vi "Get Property Values (Date Property).vi"(1 "data type":timestamp[](array[timestamp]), 5 "property":T2 {"data type" items=["Unknown"=0, "String"=23, "I32"=3, "I64"=4, "DBL"=10, "Time stamp"=30]; "object type" items=["File", "Channel Group", "Channel"]}, 7 "result references":T1[](array[typedef]), 11 "error in (no error)":errorcluster) -> (6 "property values":timestamp[](array[timestamp]), 8 "result references out":T1[](array[typedef]), 15 "error out":errorcluster)   [LabVIEW 2020, in "NI_DataFinder.lvlib"]
doc: "Determines from the result references the values of a time/date property."
uses:
  <vilib>/DataFinder/NI_DataFinder.lvlib
  <vilib>/DataFinder/DataTypes/property.ctl
  <vilib>/DataFinder/DataTypes/object type.ctl
  <vilib>/DataFinder/DataTypes/data type.ctl
  <vilib>/userdefined/DFSearchResult.ctl
  <vilib>/userdefined/NI_DataFinder Controls.lvlib
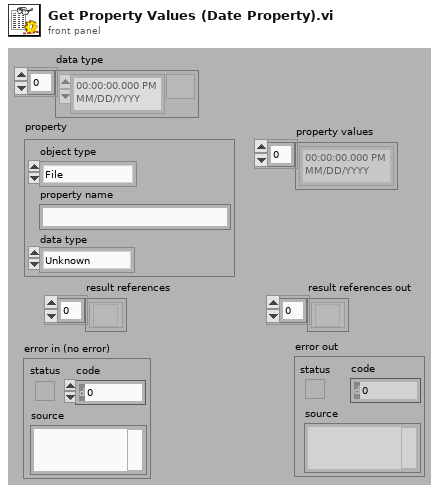
[diagram p1: front panel]
types:
  T1 = typedef "NI_DataFinder Controls.lvlib/DFSearchResult.ctl" = refnum<k20>
  T2 = typedef "NI_DataFinder.lvlib/property.ctl" = cluster{"object type":T3, "property name":string, "data type":T4}
  T3 = typedef "NI_DataFinder.lvlib/object type.ctl" = u16
  T4 = typedef "NI_DataFinder.lvlib/data type.ctl" = u16
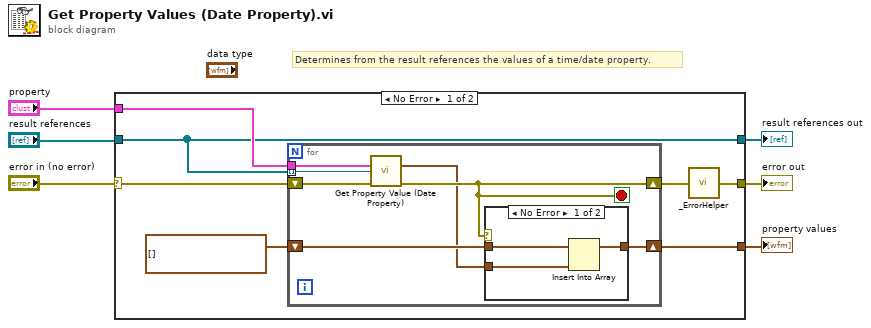
[diagram p0: block diagram]
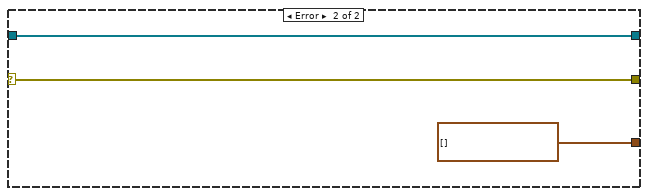
[diagram p3: hidden frame]
diagram:
  # "Determines from the result references the values of a time/date property."
  n1 = case shown="No Error" "error in (no error)" {
    selector: "error in (no error)" -> [w11 w27]
    tunnel: "result references" -> [w9 w26]
    tunnel: "property" -> [w12 _]
    tunnel: [w10 w27] -> w5
    tunnel: [w9 w26] -> w2
    tunnel: [w13 timestamp[] []] -> w1
    frame No Error {
      n2 = for {
        tunnel: w9 -> [w15] mode=indexing
        tunnel: w12 -> [w16]
        shift-right: [w18] -> w8
        shift-left: w11 -> [w14]
        shift-right: [w20] -> w13
        shift-left: timestamp[] [] -> [w19]
        stop <- w18 stop-if-true
        n3 = call <vilib>:"Get Property Value (Date Property).vi"("property"=w16, "result reference"=w15, "error in (no error)"=w14) -> ("property value"=w17:timestamp, "error out"=w18:errorcluster)  [unwired: 10 in, 1 out]
        n4 = case shown="No Error" w18 {
          tunnel: w19 -> [w23 w24]
          tunnel: [w22 w24] -> w20
          tunnel: w17 -> [w21 _]
          frame No Error {
            n5 = Insert Into Array(array=w23, new element=w21) -> (w22:timestamp[])  [unwired: 1 in]
          }
          frame Error {
          }
        }
      }
      n6 = call <vilib>:"_ErrorHelper.vi"("error IO"=w8) -> ("error out"=w10:errorcluster)
    }
    frame Error {
    }
  }
  "property values" <- w1
  "error out" <- w5
  "result references out" <- w2
